vi "ZK Create MB.vi"() -> ()   [LabVIEW 2016, in "质控单元V2.lvlib"]
uses:
  <vilib>/Plasmionique/MB Master/MB_Master_Serial/MB_Master_Serial.lvclass
  D:/Program Files (x86)/National Instruments/LabVIEW 2016/vi.lib/Plasmionique/MB Master/MB_Master/MB_Master.lvclass
  <vilib>/Plasmionique/MB Master/MB_Master_TCP/MB_Master_TCP.lvclass
  <vilib>/Plasmionique/MB Master/MB_Master/MB_Master.lvclass
  Alarm interface/Alarm interface.lvlib
panel:
  out "auto connected":bool=TRUE
  out "error out":errorcluster
  out "Connected":bool
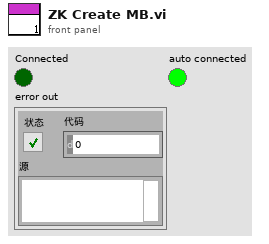
[diagram p1: front panel]
types:
  T1 = cluster{"baud rate (bps)":u32, "stop bits":u16, "parity":u16, "flow control":u16, "timeout":u32, "retries":i32}
  T2 = typedef "质控单元V2.lvlib/质控slave id.ctl" = enum16{"null", "氨氮", "总磷", "总氮", "CODMn", "CODCr"}
  T3 = cluster{"module name":string, "moduleid":i32, "sysid":i32, "content":string, "analysis":string}
  T4 = enum16{"营养盐", "V2CODMn", "新CODMn", "动力环境", "质控单元", "采配水", "其他"}
  T5 = cluster{"氨氮":bool, "总磷":bool, "总氮":bool, "CODMn":bool, "CODCr":bool, "氨氮总磷":bool, "总磷总氮":bool}
  T6 = typedef "质控单元V2.lvlib/质控仪器状态显示.ctl" = cluster{"运行模式":string, "运行状态":string, "液位状态":string, "告警状态":string, "当前流程":string, "当前步骤":string, "剩余时间":string}
  T7 = typedef "质控单元V2.lvlib/质控仪器状态.ctl" = cluster{"运行状态":enum16{"待机", "润洗", "进样", "定量", "加标", "等待取样", "排液"}, "液位状态":enum16{"无感应", "有感应"}, "告警状态":enum16{"无告警", "液位故障告警", "注射泵异常"}, "当前步骤数":u16, "当前步骤剩余时间":u16, "当前步骤具体操作":enum16{"加标", "进样", "排液", "搅拌", "定量"}, "当前流程":enum16{"待机", "进样流程", "加标流程", "排液流程"}}
  T8 = cluster{"modid":i32, "sysid":i32, "content":string, "故障详情":string}
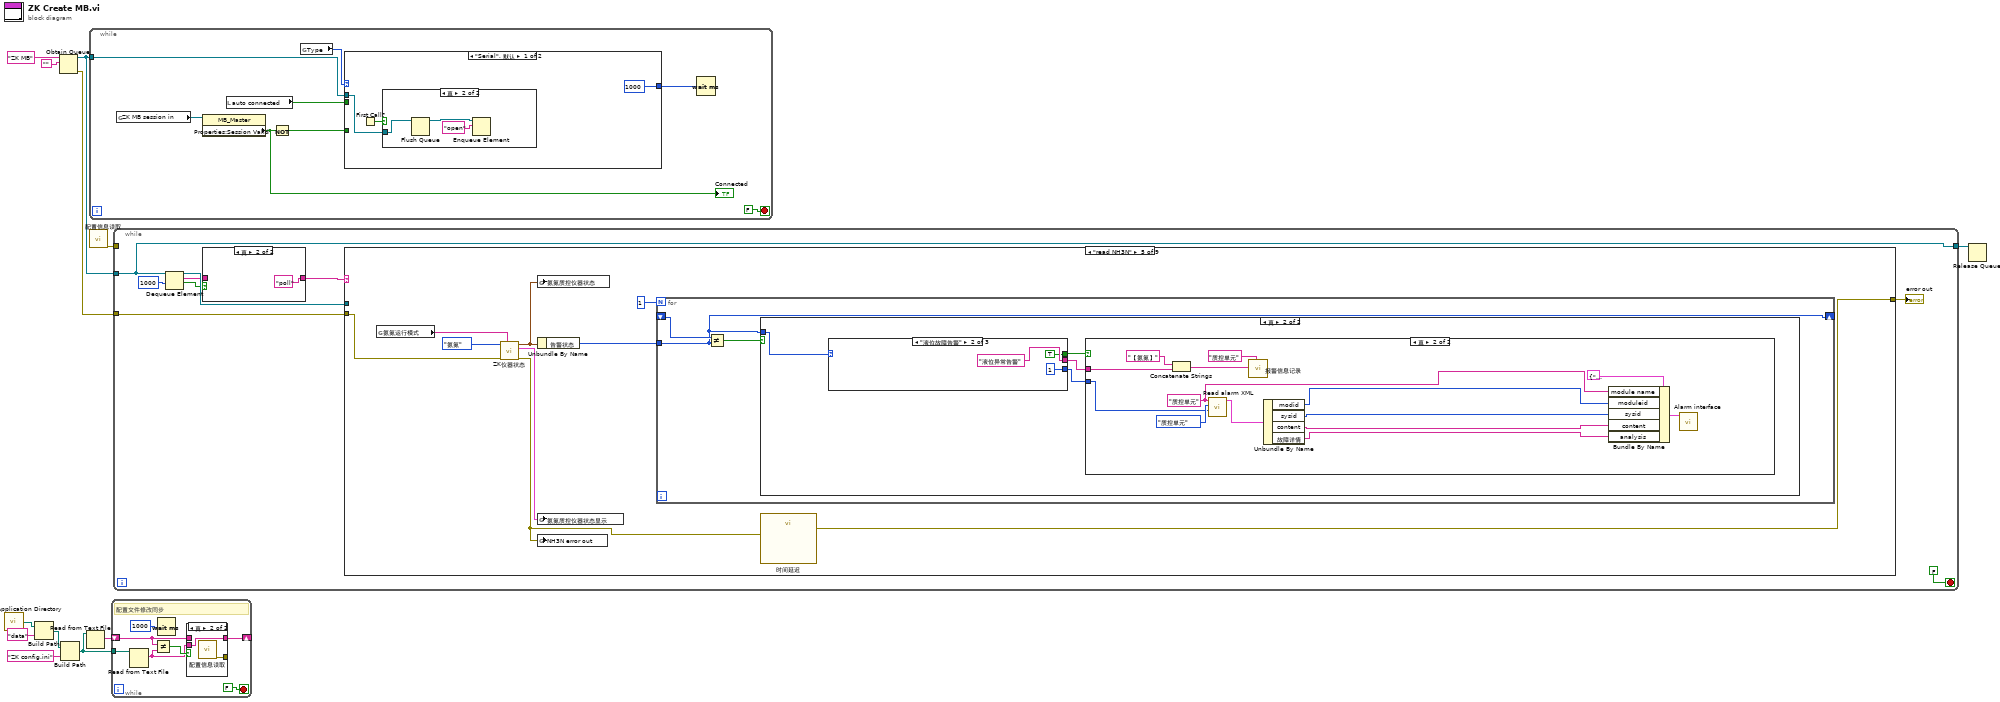
[diagram p0: block diagram]
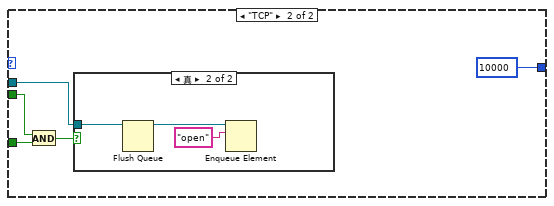
[diagram p4: hidden frame]
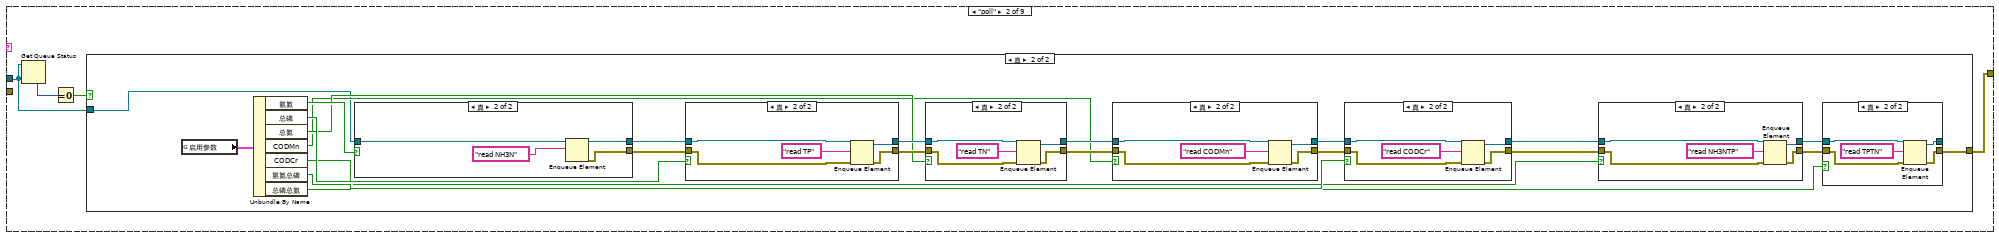
[diagram p8: hidden frame]
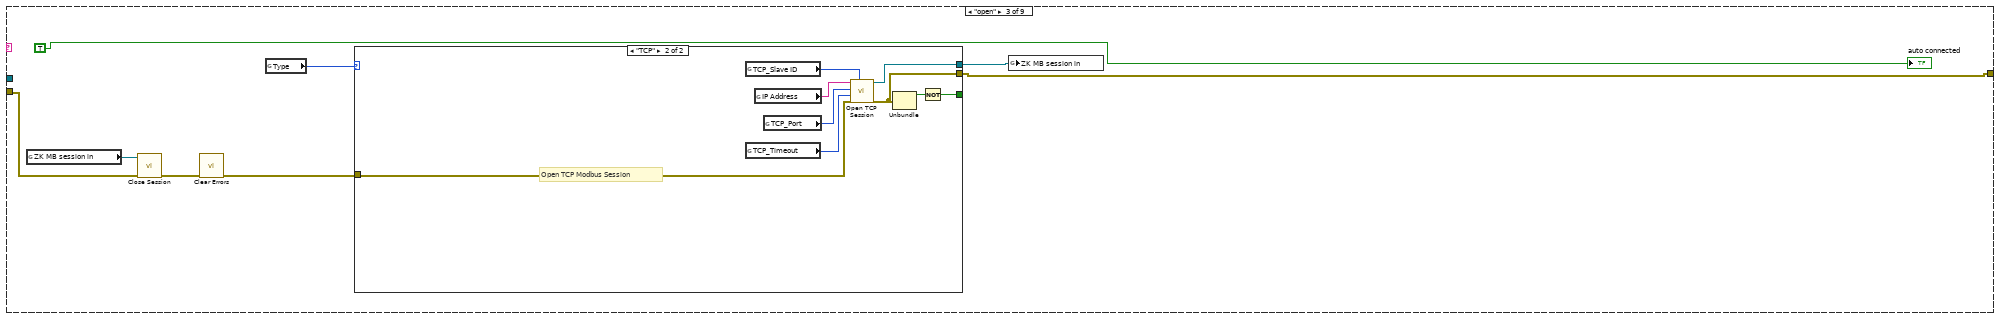
[diagram p17: hidden frame]
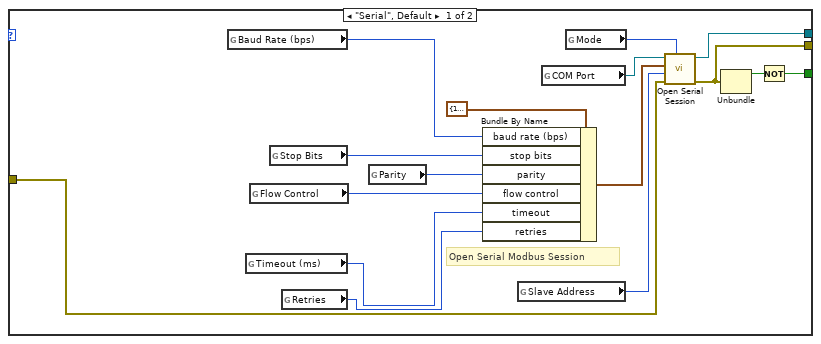
[diagram p18: hidden frame]
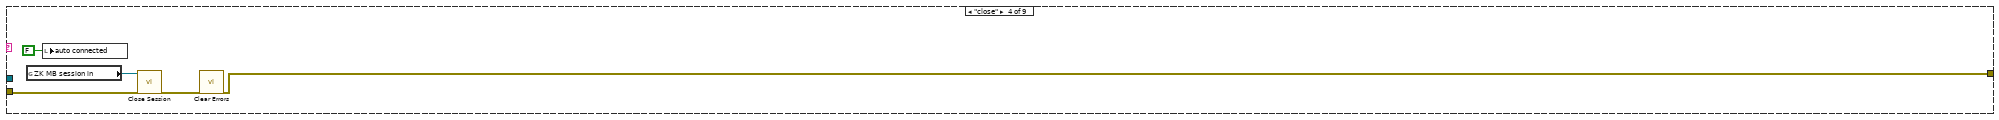
[diagram p19: hidden frame]
diagram:
  n1 = call <vilib>:"Application Directory.vi"() -> ("Application Directory"=w6:path)
  n2 = Build Path(base path=w6, name or relative path="data" ("名称或相对路径")) -> (appended path=w3:path)
  n3 = Obtain Queue(name (unnamed)="ZK MB" ("名称（未命名）"), element data type="") -> (queue out=w10:refnum<queue>, error out=w8:errorcluster)  [unwired: 3 in, 1 out]
  n4 = Build Path(base path=w3, name or relative path="ZK config.ini" ("名称或相对路径")) -> (appended path=w1:path)
  n5 = Read from Text File(file (use dialog)=w1) -> (text=w2:string)  [unwired: 3 in, 3 out]
  n6 = while {
    tunnel: w10 -> [w19]
    stop <- FALSE stop-if-true
    n7 = global read "ZK非断电保存全局变量.vi" "ZK MB session in"() -> (w16:refnum<class "MB_Master.lvclass">)
    n8 = property class="MB_Master"(reference=w16) -> ("Properties:Session Valid"=w15:bool)  [unwired: 1 in, 2 out]
    "Connected" <- w15
    n9 = local read "auto connected"() -> (w14:bool)
    n10 = Not(x=w15) -> (.not. x?=w13:bool)
    n11 = global read "ZK断电保存全局变量.vi" "Type"() -> (w20:enum16{"Serial", "TCP"})
    n12 = case shown="\"Serial\", 默认" w20 {
      tunnel: w19 -> [w23 w31]
      tunnel: [u32 1000 ("等待时间（毫秒）") u32 10000 ("等待时间（毫秒）")] -> w17
      tunnel: w13 -> [_ w29]
      tunnel: w14 -> [_ w27]
      frame "Serial", Default {
        n13 = First Call?() -> (First Call?: T/F=w22:bool)
        n14 = case shown="真" w22 {
          tunnel: w23 -> [_ w26]
          frame False {
          }
          frame True {
            n15 = Flush Queue(queue=w26) -> (queue out=w24:refnum<queue>)  [unwired: 1 in, 2 out]
            n16 = Enqueue Element(queue=w24, element="open") -> ()  [unwired: 2 in, 3 out]
          }
        }
      }
      frame "TCP" {
        n17 = And(x=w27, y=w29) -> (x .and. y?=w28:bool)
        n18 = case shown="真" w28 {
          tunnel: w31 -> [_ w33]
          frame False {
          }
          frame True {
            n19 = Flush Queue(queue=w33) -> (queue out=w32:refnum<queue>)  [unwired: 1 in, 2 out]
            n20 = Enqueue Element(queue=w32, element="open") -> ()  [unwired: 2 in, 3 out]
          }
        }
      }
    }
    n21 = Wait (ms)(milliseconds to wait=w17) -> ()  [unwired: 1 out]
  }
  n22 = call "配置信息读取.vi"() -> ("error out"=w7:errorcluster)  [unwired: 11 in]
  n23 = while {
    shift-right: [w39] -> _
    shift-left: w2 -> [w37]
    tunnel: w1 -> [w41]
    stop <- FALSE stop-if-true
    # "配置文件修改同步"
    n24 = Read from Text File(file (use dialog)=w41) -> (text=w38:string)  [unwired: 3 in, 3 out]
    n25 = Not Equal?(x=w37, y=w38) -> (x != y?=w40:bool)
    n26 = Wait (ms)(milliseconds to wait=u32 1000 ("等待时间（毫秒）")) -> ()  [unwired: 1 out]
    n27 = case shown="真" w40 {
      tunnel: [w42 w44] -> w39
      tunnel: w38 -> [_ w44]
      tunnel: w37 -> [w42 _]
      tunnel: [_ w43] -> _
      frame False {
      }
      frame True {
        n28 = call "配置信息读取.vi"() -> ("error out"=w43:errorcluster)  [unwired: 11 in]
      }
    }
  }
  n29 = while {
    tunnel: w10 -> [w50]
    tunnel: [w50] -> w9
    tunnel: w8 -> [w45]
    tunnel: w7 -> [_]
    stop <- FALSE stop-if-true
    n30 = Dequeue Element(queue=w50, timeout in ms (-1)=1000 ("超时毫秒(-1)")) -> (queue out=w51:refnum<queue>, element=w47:string, timed out?=w48:bool)  [unwired: 1 in, 1 out]
    n31 = case shown="真" w48 {
      tunnel: w47 -> [w54 _]
      tunnel: [w54 "poll"] -> w46
      frame False {
      }
      frame True {
      }
    }
    n32 = case shown="\"read NH3N\"" w46 {
      tunnel: [w56 w60 w132 w165 w173 w209 w245 w281 w317] -> w52
      tunnel: w45 -> [w56 _ w131 w166 w176 w212 w248 w284 w320]
      tunnel: w51 -> [_ w59 _ _ _ _ _ _ _]
      frame Default {
      }
      frame "poll" {
        n33 = Get Queue Status(queue=w59) -> (# elements in queue=w58:i32)  [unwired: 2 in, 7 out]
        n34 = Equal To 0?(x=w58) -> (x = 0?=w57:bool)
        n35 = case shown="真" w57 {
          tunnel: [_ w66] -> w60
          tunnel: w59 -> [_ w61]
          frame False {
          }
          frame True {
            n36 = global read "ZK断电保存全局变量.vi" "启用参数"() -> (w74:T5)
            n37 = Unbundle By Name(w74) -> ("氨氮"=w73:bool, "总磷"=w72:bool, "总氮"=w71:bool, "CODMn"=w65:bool, "CODCr"=w64:bool, "氨氮总磷"=w63:bool, "总磷总氮"=w62:bool)
            n38 = case shown="真" w73 {
              tunnel: w61 -> [w125 w129]
              tunnel: [w125 w128] -> w82
              tunnel: [_ w127] -> w81
              frame False {
              }
              frame True {
                n39 = Enqueue Element(queue=w129, element="read NH3N") -> (queue out=w128:refnum<queue>, error out=w127:errorcluster)  [unwired: 2 in, 1 out]
              }
            }
            n40 = case shown="真" w72 {
              tunnel: w82 -> [w119 w124]
              tunnel: w81 -> [w118 w123]
              tunnel: [w119 w121] -> w80
              tunnel: [w118 w120] -> w77
              frame False {
              }
              frame True {
                n41 = Enqueue Element(queue=w124, element="read TP", error in (no error)=w123) -> (queue out=w121:refnum<queue>, error out=w120:errorcluster)  [unwired: 1 in, 1 out]
              }
            }
            n42 = case shown="真" w71 {
              tunnel: w80 -> [w112 w116]
              tunnel: [w112 w115] -> w70
              tunnel: w77 -> [w111 w114]
              tunnel: [w111 w113] -> w69
              frame False {
              }
              frame True {
                n43 = Enqueue Element(queue=w116, element="read TN", error in (no error)=w114) -> (queue out=w115:refnum<queue>, error out=w113:errorcluster)  [unwired: 1 in, 1 out]
              }
            }
            n44 = case shown="真" w65 {
              tunnel: w70 -> [w91 w95]
              tunnel: [w91 w94] -> w78
              tunnel: w69 -> [w90 w93]
              tunnel: [w90 w92] -> w75
              frame False {
              }
              frame True {
                n45 = Enqueue Element(queue=w95, element="read CODMn", error in (no error)=w93) -> (queue out=w94:refnum<queue>, error out=w92:errorcluster)  [unwired: 1 in, 1 out]
              }
            }
            n46 = case shown="真" w64 {
              tunnel: w78 -> [w84 w89]
              tunnel: w75 -> [w83 w88]
              tunnel: [w83 w86] -> w67
              tunnel: [w84 w85] -> w68
              frame False {
              }
              frame True {
                n47 = Enqueue Element(queue=w89, element="read CODCr", error in (no error)=w88) -> (queue out=w85:refnum<queue>, error out=w86:errorcluster)  [unwired: 1 in, 1 out]
              }
            }
            n48 = case shown="真" w63 {
              tunnel: w68 -> [w105 w109]
              tunnel: [w105 w108] -> w79
              tunnel: w67 -> [w104 w107]
              tunnel: [w104 w106] -> w76
              frame False {
              }
              frame True {
                n49 = Enqueue Element(queue=w109, element="read NH3NTP", error in (no error)=w107) -> (queue out=w108:refnum<queue>, error out=w106:errorcluster)  [unwired: 1 in, 1 out]
              }
            }
            n50 = case shown="真" w62 {
              tunnel: w79 -> [w98 w102]
              tunnel: [w98 w101] -> _
              tunnel: w76 -> [w97 w100]
              tunnel: [w97 w99] -> w66
              frame False {
              }
              frame True {
                n51 = Enqueue Element(queue=w102, element="read TPTN", error in (no error)=w100) -> (queue out=w101:refnum<queue>, error out=w99:errorcluster)  [unwired: 1 in, 1 out]
              }
            }
          }
        }
      }
      frame "open" {
        n52 = global read "ZK非断电保存全局变量.vi" "ZK MB session in"() -> (w134:refnum<class "MB_Master.lvclass">)
        n53 = call-dynamic "Close Session.vi"("error in (no error)"=w131, "MB session in"=w134) -> ("error out"=w136:errorcluster)  [unwired: 9 in]
        n54 = call <vilib>:"Clear Errors.vi"("error in (no error)"=w136) -> ("error out"=w137:errorcluster)  [unwired: 5 in, 1 out]
        n55 = global read "ZK断电保存全局变量.vi" "Type"() -> (w135:enum16{"Serial", "TCP"})
        n56 = case shown="\"TCP\"" w135 {
          tunnel: [w151 w158] -> w133
          tunnel: [w150 w159] -> w132
          tunnel: [w148 w160] -> _
          tunnel: w137 -> [w147 w162]
          frame "Serial", Default {
            # "Open Serial Modbus Session"
            n57 = global read "ZK断电保存全局变量.vi" "Baud Rate (bps)"() -> (w143:u32)
            n58 = global read "ZK断电保存全局变量.vi" "Timeout (ms)"() -> (w139:u32)
            n59 = global read "ZK断电保存全局变量.vi" "Flow Control"() -> (w140:u16)
            n60 = global read "ZK断电保存全局变量.vi" "Stop Bits"() -> (w142:u16)
            n61 = global read "ZK断电保存全局变量.vi" "Retries"() -> (w138:i32)
            n62 = global read "ZK断电保存全局变量.vi" "Parity"() -> (w141:u16)
            n63 = Bundle By Name(cluster=T1 {"baud rate (bps)"=19200, "stop bits"=10, "parity"=0, "flow control"=0, "timeout"=1000, "retries"=1} ("Serial Config"), "baud rate (bps)"=w143, "stop bits"=w142, "parity"=w141, "flow control"=w140, "timeout"=w139, "retries"=w138) -> (w152:T1)
            n64 = global read "ZK断电保存全局变量.vi" "Slave Address"() -> (w144:u8)
            n65 = global read "ZK断电保存全局变量.vi" "COM Port"() -> (w145:refnum<visa-resource-name>)
            n66 = global read "ZK断电保存全局变量.vi" "Mode"() -> (w146:enum16{"RTU", "ASCII"})
            n67 = call <vilib>:"Open Serial Session.vi"("Mode (RTU)"=w146, "Error in"=w147, "Slave ID"=w144, "Serial Config"=w152, "VISA Resource"=w145) -> ("Error out"=w150:errorcluster, "MB_Serial session"=w151:refnum<class "MB_Master_Serial.lvclass">)  [unwired: 5 in]
            n68 = Unbundle(w150) -> ("status"=w149:bool)  [unwired: 2 out]
            n69 = Not(x=w149) -> (.not. x?=w148:bool)
          }
          frame "TCP" {
            # "Open TCP Modbus Session"
            n70 = global read "ZK断电保存全局变量.vi" "TCP_Slave ID"() -> (w157:u8)
            n71 = global read "ZK断电保存全局变量.vi" "TCP_Timeout"() -> (w154:i32)
            n72 = global read "ZK断电保存全局变量.vi" "IP Address"() -> (w156:string)
            n73 = global read "ZK断电保存全局变量.vi" "TCP_Port"() -> (w155:u16)
            n74 = call <vilib>:"Open TCP Session.vi"("Slave ID (255)"=w157, "error in (no error)"=w162, "Timeout (10000)"=w154, "Port (502)"=w155, "IP Address"=w156) -> ("error out"=w159:errorcluster, "MB_TCP session"=w158:refnum<class "MB_Master_TCP.lvclass">)  [unwired: 5 in]
            n75 = Unbundle(w159) -> ("status"=w161:bool)  [unwired: 2 out]
            n76 = Not(x=w161) -> (.not. x?=w160:bool)
          }
        }
        n77 = global write "ZK非断电保存全局变量.vi" "ZK MB session in"(w133) -> ()
        "auto connected" <- TRUE
      }
      frame "close" {
        n78 = global read "ZK非断电保存全局变量.vi" "ZK MB session in"() -> (w164:refnum<class "MB_Master.lvclass">)
        n79 = local write "auto connected"(FALSE ("auto connected")) -> ()
        n80 = call-dynamic "Close Session.vi"("error in (no error)"=w166, "MB session in"=w164) -> ("error out"=w167:errorcluster)  [unwired: 9 in]
        n81 = call <vilib>:"Clear Errors.vi"("error in (no error)"=w167) -> ("error out"=w165:errorcluster)  [unwired: 5 in, 1 out]
      }
      frame "read NH3N" {
        n82 = global read "ZK非断电保存全局变量.vi" "氨氮运行模式"() -> (w168:string)
        n83 = call "ZK仪器状态.vi"("运行模式"=w168, "error in (no error)"=w176, "Slave ID"=质控slave_id."氨氮") -> ("error out"=w174:errorcluster, "质控仪器状态显示"=w172:T6, "质控仪器状态"=w171:T7)  [unwired: 6 in]
        n84 = global write "ZK非断电保存全局变量.vi" "氨氮质控仪器状态"(w171) -> ()
        n85 = Unbundle By Name(w171) -> ("告警状态"=w169:enum16{"无告警", "液位故障告警", "注射泵异常"})
        n86 = global write "ZK非断电保存全局变量.vi" "氨氮质控仪器状态显示"(w172) -> ()
        n87 = global write "ZK非断电保存全局变量.vi" "NH3N error out"(w174) -> ()
        n88 = for {
          N: 1 -> [_]
          shift-right: [w178] -> _
          shift-left: _ -> [w179]
          tunnel: w169 -> [w178]
          n89 = Not Equal?(x=w179, y=w178) -> (x != y?=w177:bool)
          n90 = case shown="真" w177 {
            tunnel: w178 -> [_ w183]
            frame False {
            }
            frame True {
              n91 = case shown="\"液位故障告警\"" w183 {
                tunnel: [_ "液位异常告警" ("字符串") "柱塞泵故障告警" ("字符串")] -> w181
                tunnel: [_ TRUE TRUE] -> w182
                tunnel: [_ 1 ("code") 2 ("code")] -> w180
                frame "无告警", Default {
                }
                frame "液位故障告警" {
                }
                frame "注射泵异常" {
                }
              }
              n92 = case shown="真" w182 {
                tunnel: w181 -> [_ w202]
                tunnel: w180 -> [_ w195]
                frame False {
                }
                frame True {
                  w198 = "质控单元" ("模块名称")
                  n93 = Concatenate Strings("【氨氮】" ("字符串"), w202) -> (w200:string)
                  n94 = call "Read alarm XML.vi"("告警代码"=w195, "模块常量"=T4."质控单元", "模块名称"=w198) -> ("报警"=w194:T8)  [unwired: 8 in]
                  n95 = call "报警信息记录.vi"("参数"="质控单元", "报警信息"=w200) -> ()  [unwired: 9 in, 1 out]
                  n96 = Unbundle By Name(w194) -> ("modid"=w193:i32, "sysid"=w192:i32, "content"=w191:string, "故障详情"=w190:string)
                  n97 = Bundle By Name(cluster=T3 {"module name"="", "moduleid"=0, "sysid"=0, "content"="", "analysis"=""} ("簇"), "module name"=w198, "moduleid"=w193, "sysid"=w192, "content"=w191, "analysis"=w190) -> (w196:T3)
                  n98 = call "Alarm interface.vi"("簇"=w196) -> ()  [unwired: 10 in, 1 out]
                }
              }
            }
          }
        }
        n99 = call "时间延迟"("error in (no error)"=w174) -> ("error out"=w173:errorcluster)  [unwired: 10 in]
      }
      frame "read TP" {
        n100 = global read "ZK非断电保存全局变量.vi" "总磷运行模式"() -> (w204:string)
        n101 = call "ZK仪器状态.vi"("运行模式"=w204, "error in (no error)"=w212, "Slave ID"=质控slave_id."总磷") -> ("error out"=w210:errorcluster, "质控仪器状态显示"=w208:T6, "质控仪器状态"=w207:T7)  [unwired: 6 in]
        n102 = global write "ZK非断电保存全局变量.vi" "总磷质控仪器状态"(w207) -> ()
        n103 = Unbundle By Name(w207) -> ("告警状态"=w206:enum16{"无告警", "液位故障告警", "注射泵异常"})
        n104 = global write "ZK非断电保存全局变量.vi" "总磷质控仪器状态显示"(w208) -> ()
        n105 = global write "ZK非断电保存全局变量.vi" "tp error out"(w210) -> ()
        n106 = for {
          N: 1 -> [_]
          shift-right: [w214] -> _
          shift-left: _ -> [w215]
          tunnel: w206 -> [w214]
          n107 = Not Equal?(x=w215, y=w214) -> (x != y?=w213:bool)
          n108 = case shown="真" w213 {
            tunnel: w214 -> [_ w219]
            frame False {
            }
            frame True {
              n109 = case shown="\"液位故障告警\"" w219 {
                tunnel: [_ "液位异常告警" ("字符串") "柱塞泵故障告警" ("字符串")] -> w217
                tunnel: [_ TRUE TRUE] -> w218
                tunnel: [_ 1 ("code") 2 ("code")] -> w216
                frame "无告警", Default {
                }
                frame "液位故障告警" {
                }
                frame "注射泵异常" {
                }
              }
              n110 = case shown="真" w218 {
                tunnel: w217 -> [_ w238]
                tunnel: w216 -> [_ w231]
                frame False {
                }
                frame True {
                  w234 = "质控单元" ("模块名称")
                  n111 = Concatenate Strings("【总磷】" ("字符串"), w238) -> (w236:string)
                  n112 = call "Read alarm XML.vi"("告警代码"=w231, "模块常量"=T4."质控单元", "模块名称"=w234) -> ("报警"=w230:T8)  [unwired: 8 in]
                  n113 = call "报警信息记录.vi"("参数"="质控单元", "报警信息"=w236) -> ()  [unwired: 9 in, 1 out]
                  n114 = Unbundle By Name(w230) -> ("modid"=w229:i32, "sysid"=w228:i32, "content"=w227:string, "故障详情"=w226:string)
                  n115 = Bundle By Name(cluster=T3 {"module name"="", "moduleid"=0, "sysid"=0, "content"="", "analysis"=""} ("簇"), "module name"=w234, "moduleid"=w229, "sysid"=w228, "content"=w227, "analysis"=w226) -> (w232:T3)
                  n116 = call "Alarm interface.vi"("簇"=w232) -> ()  [unwired: 10 in, 1 out]
                }
              }
            }
          }
        }
        n117 = call "时间延迟2"("error in (no error)"=w210) -> ("error out"=w209:errorcluster)  [unwired: 10 in]
      }
      frame "read TN" {
        n118 = global read "ZK非断电保存全局变量.vi" "总氮运行模式"() -> (w240:string)
        n119 = call "ZK仪器状态.vi"("运行模式"=w240, "error in (no error)"=w248, "Slave ID"=质控slave_id."总氮") -> ("error out"=w246:errorcluster, "质控仪器状态显示"=w244:T6, "质控仪器状态"=w243:T7)  [unwired: 6 in]
        n120 = global write "ZK非断电保存全局变量.vi" "总氮质控仪器状态"(w243) -> ()
        n121 = Unbundle By Name(w243) -> ("告警状态"=w242:enum16{"无告警", "液位故障告警", "注射泵异常"})
        n122 = global write "ZK非断电保存全局变量.vi" "总氮质控仪器状态显示"(w244) -> ()
        n123 = global write "ZK非断电保存全局变量.vi" "tn error out"(w246) -> ()
        n124 = for {
          N: 1 -> [_]
          shift-right: [w250] -> _
          shift-left: _ -> [w251]
          tunnel: w242 -> [w250]
          n125 = Not Equal?(x=w251, y=w250) -> (x != y?=w249:bool)
          n126 = case shown="真" w249 {
            tunnel: w250 -> [_ w255]
            frame False {
            }
            frame True {
              n127 = case shown="\"液位故障告警\"" w255 {
                tunnel: [_ "液位异常告警" ("字符串") "柱塞泵故障告警" ("字符串")] -> w253
                tunnel: [_ TRUE TRUE] -> w254
                tunnel: [_ 1 ("code") 2 ("code")] -> w252
                frame "无告警", Default {
                }
                frame "液位故障告警" {
                }
                frame "注射泵异常" {
                }
              }
              n128 = case shown="真" w254 {
                tunnel: w253 -> [_ w274]
                tunnel: w252 -> [_ w267]
                frame False {
                }
                frame True {
                  w270 = "质控单元" ("模块名称")
                  n129 = Concatenate Strings("【总氮】" ("字符串"), w274) -> (w272:string)
                  n130 = call "Read alarm XML.vi"("告警代码"=w267, "模块常量"=T4."质控单元", "模块名称"=w270) -> ("报警"=w266:T8)  [unwired: 8 in]
                  n131 = Unbundle By Name(w266) -> ("modid"=w265:i32, "sysid"=w264:i32, "content"=w263:string, "故障详情"=w262:string)
                  n132 = call "报警信息记录.vi"("参数"="质控单元", "报警信息"=w272) -> ()  [unwired: 9 in, 1 out]
                  n133 = Bundle By Name(cluster=T3 {"module name"="", "moduleid"=0, "sysid"=0, "content"="", "analysis"=""} ("簇"), "module name"=w270, "moduleid"=w265, "sysid"=w264, "content"=w263, "analysis"=w262) -> (w268:T3)
                  n134 = call "Alarm interface.vi"("簇"=w268) -> ()  [unwired: 10 in, 1 out]
                }
              }
            }
          }
        }
        n135 = call "时间延迟3"("error in (no error)"=w246) -> ("error out"=w245:errorcluster)  [unwired: 10 in]
      }
      frame "read CODMn" {
        n136 = global read "ZK非断电保存全局变量.vi" "CODMn运行模式"() -> (w276:string)
        n137 = call "ZK仪器状态.vi"("运行模式"=w276, "error in (no error)"=w284, "Slave ID"=质控slave_id."CODMn") -> ("error out"=w282:errorcluster, "质控仪器状态显示"=w280:T6, "质控仪器状态"=w279:T7)  [unwired: 6 in]
        n138 = global write "ZK非断电保存全局变量.vi" "CODMn质控仪器状态"(w279) -> ()
        n139 = Unbundle By Name(w279) -> ("告警状态"=w278:enum16{"无告警", "液位故障告警", "注射泵异常"})
        n140 = global write "ZK非断电保存全局变量.vi" "CODMn质控仪器状态显示"(w280) -> ()
        n141 = global write "ZK非断电保存全局变量.vi" "CODMn error out"(w282) -> ()
        n142 = for {
          N: 1 -> [_]
          shift-right: [w286] -> _
          shift-left: _ -> [w287]
          tunnel: w278 -> [w286]
          n143 = Not Equal?(x=w287, y=w286) -> (x != y?=w285:bool)
          n144 = case shown="真" w285 {
            tunnel: w286 -> [_ w291]
            frame False {
            }
            frame True {
              n145 = case shown="\"无告警\", 默认" w291 {
                tunnel: [_ "液位异常告警" ("字符串") "柱塞泵故障告警" ("字符串")] -> w289
                tunnel: [_ TRUE TRUE] -> w290
                tunnel: [_ 1 ("code") 2 ("code")] -> w288
                frame "无告警", Default {
                }
                frame "液位故障告警" {
                }
                frame "注射泵异常" {
                }
              }
              n146 = case shown="真" w290 {
                tunnel: w289 -> [_ w310]
                tunnel: w288 -> [_ w303]
                frame False {
                }
                frame True {
                  w306 = "质控单元" ("模块名称")
                  n147 = call "Read alarm XML.vi"("告警代码"=w303, "模块常量"=T4."质控单元", "模块名称"=w306) -> ("报警"=w302:T8)  [unwired: 8 in]
                  n148 = Concatenate Strings("【CODMn】" ("字符串"), w310) -> (w308:string)
                  n149 = Unbundle By Name(w302) -> ("modid"=w301:i32, "sysid"=w300:i32, "content"=w299:string, "故障详情"=w298:string)
                  n150 = call "报警信息记录.vi"("参数"="质控单元", "报警信息"=w308) -> ()  [unwired: 9 in, 1 out]
                  n151 = Bundle By Name(cluster=T3 {"module name"="", "moduleid"=0, "sysid"=0, "content"="", "analysis"=""} ("簇"), "module name"=w306, "moduleid"=w301, "sysid"=w300, "content"=w299, "analysis"=w298) -> (w304:T3)
                  n152 = call "Alarm interface.vi"("簇"=w304) -> ()  [unwired: 10 in, 1 out]
                }
              }
            }
          }
        }
        n153 = call "时间延迟4"("error in (no error)"=w282) -> ("error out"=w281:errorcluster)  [unwired: 10 in]
      }
      frame "read CODCr" {
        n154 = global read "ZK非断电保存全局变量.vi" "CODCr运行模式"() -> (w312:string)
        n155 = call "ZK仪器状态.vi"("运行模式"=w312, "error in (no error)"=w320, "Slave ID"=质控slave_id."CODCr") -> ("error out"=w318:errorcluster, "质控仪器状态显示"=w316:T6, "质控仪器状态"=w315:T7)  [unwired: 6 in]
        n156 = global write "ZK非断电保存全局变量.vi" "CODCr质控仪器状态"(w315) -> ()
        n157 = Unbundle By Name(w315) -> ("告警状态"=w314:enum16{"无告警", "液位故障告警", "注射泵异常"})
        n158 = global write "ZK非断电保存全局变量.vi" "CODcr质控仪器状态显示"(w316) -> ()
        n159 = global write "ZK非断电保存全局变量.vi" "CODCr error out"(w318) -> ()
        n160 = for {
          N: 1 -> [_]
          shift-right: [w322] -> _
          shift-left: _ -> [w323]
          tunnel: w314 -> [w322]
          n161 = Not Equal?(x=w323, y=w322) -> (x != y?=w321:bool)
          n162 = case shown="真" w321 {
            tunnel: w322 -> [_ w327]
            frame False {
            }
            frame True {
              n163 = case shown="\"注射泵异常\"" w327 {
                tunnel: [_ "液位异常告警" ("字符串") "柱塞泵故障告警" ("字符串")] -> w326
                tunnel: [_ TRUE TRUE] -> w325
                tunnel: [_ 1 ("元素") 2 ("元素")] -> w324
                frame "无告警", Default {
                }
                frame "液位故障告警" {
                }
                frame "注射泵异常" {
                }
              }
              n164 = case shown="真" w325 {
                tunnel: w326 -> [_ w340]
                tunnel: w324 -> [_ w335]
                frame False {
                }
                frame True {
                  w336 = "质控单元" ("模块名称")
                  n165 = call "Read alarm XML.vi"("告警代码"=w335, "模块常量"=T4."质控单元", "模块名称"=w336) -> ("报警"=w332:T8)  [unwired: 8 in]
                  n166 = Concatenate Strings("【CODCr】" ("字符串"), w340) -> (w338:string)
                  n167 = Unbundle By Name(w332) -> ("modid"=w331:i32, "sysid"=w330:i32, "content"=w329:string, "故障详情"=w328:string)
                  n168 = call "报警信息记录.vi"("参数"="质控单元", "报警信息"=w338) -> ()  [unwired: 9 in, 1 out]
                  n169 = Bundle By Name(cluster=T3 {"module name"="", "moduleid"=0, "sysid"=0, "content"="", "analysis"=""} ("簇"), "module name"=w336, "moduleid"=w331, "sysid"=w330, "content"=w329, "analysis"=w328) -> (w333:T3)
                  n170 = call "Alarm interface.vi"("簇"=w333) -> ()  [unwired: 10 in, 1 out]
                }
              }
            }
          }
        }
        n171 = call "时间延迟5"("error in (no error)"=w318) -> ("error out"=w317:errorcluster)  [unwired: 10 in]
      }
    }
    "error out" <- w52
  }
  n172 = Release Queue(queue=w9) -> ()  [unwired: 2 in, 3 out]
